vi "Save as Text.vi"(8 "error in":errorcluster, 10 "file path (use dialog)":path, 11 "array":dbl[][](array[numeric])) -> (0 "error out":errorcluster)   [LabVIEW 2018]
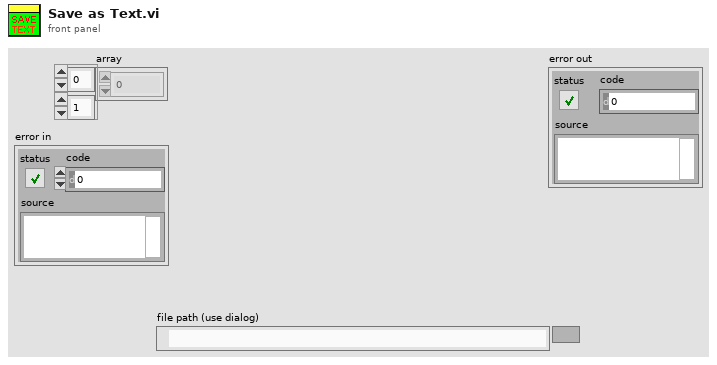
[diagram p1: front panel]
types:
  T1 = enum16{"open", "replace", "create", "open or create", "replace or create", "replace or create with confirmation"}
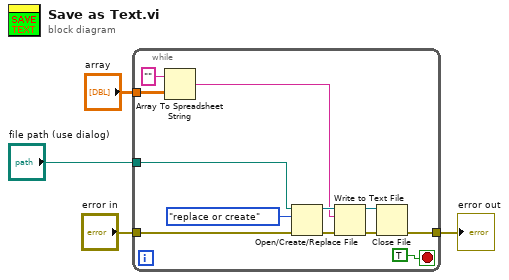
[diagram p0: block diagram]
diagram:
  n1 = while {
    tunnel: [w13] -> w1
    tunnel: "array" -> [w9]
    tunnel: "error in" -> [w8]
    tunnel: "file path (use dialog)" -> [w7]
    stop <- TRUE stop-if-true
    n2 = Array To Spreadsheet String(array=w9, 3:"" ("format string")) -> (spreadsheet string=w10:string)  [unwired: 1 in]
    n3 = Open/Create/Replace File(file path (use dialog)=w7, error in=w8, operation (0:open)=T1."replace or create") -> (refnum out=w12:refnum<file>, error out=w15:errorcluster)  [unwired: 3 in, 1 out]
    n4 = Write to Text File(file (use dialog)=w12, text=w10, error in=w15) -> (refnum out=w11:refnum<file>, error out=w14:errorcluster)  [unwired: 1 in, 1 out]
    n5 = Close File(refnum=w11, error in=w14) -> (error out=w13:errorcluster)  [unwired: 1 out]
  }
  "error out" <- w1
